vi "Main_State.vi"() -> ()   [LabVIEW 2017]
doc: "This sample project is built upon the standard state machine template and shows how you could create an application that acquires, analyzes, and presents data. It includes functionality for presenting configuration dialogs, preserving settings between executions, loading and saving data, as well as exporting graph images and text files.\n\nIt is most appropriate for data that is acquired instantly as it does not allow for screen updates mid acquisition nor does it allow for continuous streaming to disk."
uses:
  controls/State.ctl
  controls/Data.ctl
  controls/UI References.ctl
  controls/User Specified Data.ctl
  controls/HW Configuration.ctl
  controls/Analysis Configuration.ctl
  controls/New Data Behavior.ctl
  controls/Signal Configuration.ctl
  controls/TCP Multiple Connections State.ctl
  controls/TCP Multiple Connections Data.ctl
  <extravilib>/ChannelInstances/Event Messenger-str/Instantiate.vi
  <extravilib>/ChannelInstances/Event Messenger-str/))Channel.vi
  <extravilib>/ChannelInstances/Event Messenger-c(a[.](str),t'Data.ctl')/Instantiate.vi
  <extravilib>/ChannelInstances/Event Messenger-c(a[.](str),t'Data.ctl')/))Channel.vi
  subVIs/Settings Dialog.vi
  <extravilib>/ChannelInstances/Event Messenger-str.lvlib
  <extravilib>/ChannelInstances/Event Messenger-c(a[.](str),t'Data.ctl').lvlib
panel:
  out "# of Connections":i32
  in  "Settings":bool
  in  "Snapshot":bool
  in  "Analyze":bool
  in  "Clear":bool
  in  "Exit":bool
  in  "Acquire":bool
  in  "Export":bool
  in  "Save Data":bool
  in  "Load Data":bool
  out "Status Bar":string
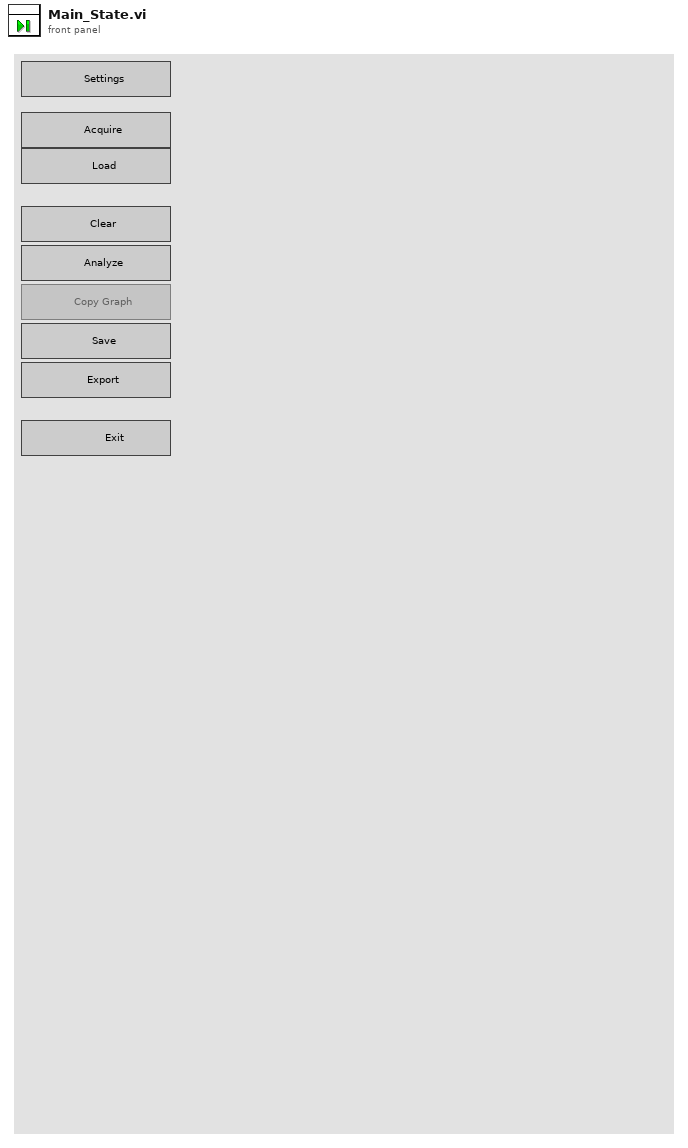
[diagram p1: front panel]
types:
  T1 = typedef "TCP Multiple Connections Data.ctl" = cluster{"Clients":refnum<k5>[], "Listener":refnum<k5>}
  T2 = typedef "TCP Multiple Connections State.ctl" = enum16{"Initialize", "Status Check", "Send Data", "Stop"}
  T3 = typedef "Data.ctl" = cluster{"UI References":T4, "User Specified":T5}
  T4 = typedef "UI References.ctl" = cluster{"Exit Ref":refnum<vi>, "Save Ref":refnum<vi>, "Open Ref":refnum<vi>, "Export Ref":refnum<vi>, "Acquire Ref":refnum<vi>, "Configure Ref":refnum<vi>, "Graph Ref":refnum<vi>, "Clear Ref":refnum<vi>, "Analyze Ref":refnum<vi>, "Status Ref":refnum<vi>, "Snapshot Ref":refnum<vi>}
  T5 = typedef "User Specified Data.ctl" = cluster{"Hardware Configuration":T6, "Analysis Configuration":T7, "Signal Type":enum16{"Single Chirp", "From Excel"}, "New Data Behavior":T8, "Signal Configuration":T9, "Waveform File":string, "Save Location":string}
  T6 = typedef "HW Configuration.ctl" = cluster{"Signal Channel":tag, "Response Channel":tag, "Trigger Channel":tag, "Number of Acquisitions":dbl}
  T7 = typedef "Analysis Configuration.ctl" = cluster{"Statistics":bool}
  T8 = typedef "New Data Behavior.ctl" = enum16{"Replace", "Overlay", "Append"}
  T9 = typedef "Signal Configuration.ctl" = cluster{"Chirp Amplitude":dbl, "I/O Limit":dbl, "Sample Rate":dbl, "Chirp Duration (s)":dbl, "Upper Frequency":dbl, "Lower Frequency":dbl, "Windowing":enum16{"None", "Exponential", "Flat top", "Hamming", "Hanning", "Kaiser-Bessel", "Rectangular"}}
  T10 = typedef "State.ctl" = enum16{"Initialize", "Wait for Event", "Update UI", "Configure", "Acquire", "Load Data", "Save Data", "Clear Data", "Export Data", "Analyze", "Copy Graph", "Exit"}
  T11 = enum16{"Standard", "Buffered", "CRLF", "Immediate"}
  T12 = typedef "Event Messenger-str.lvlib/))Channel.ctl" = refnum<queue>
  T13 = cluster{"Event message":string[], "User Specified Data":T3}
  T14 = typedef "Event Messenger-c(a[.](str),t'Data.ctl').lvlib/))Channel.ctl" = refnum<queue>
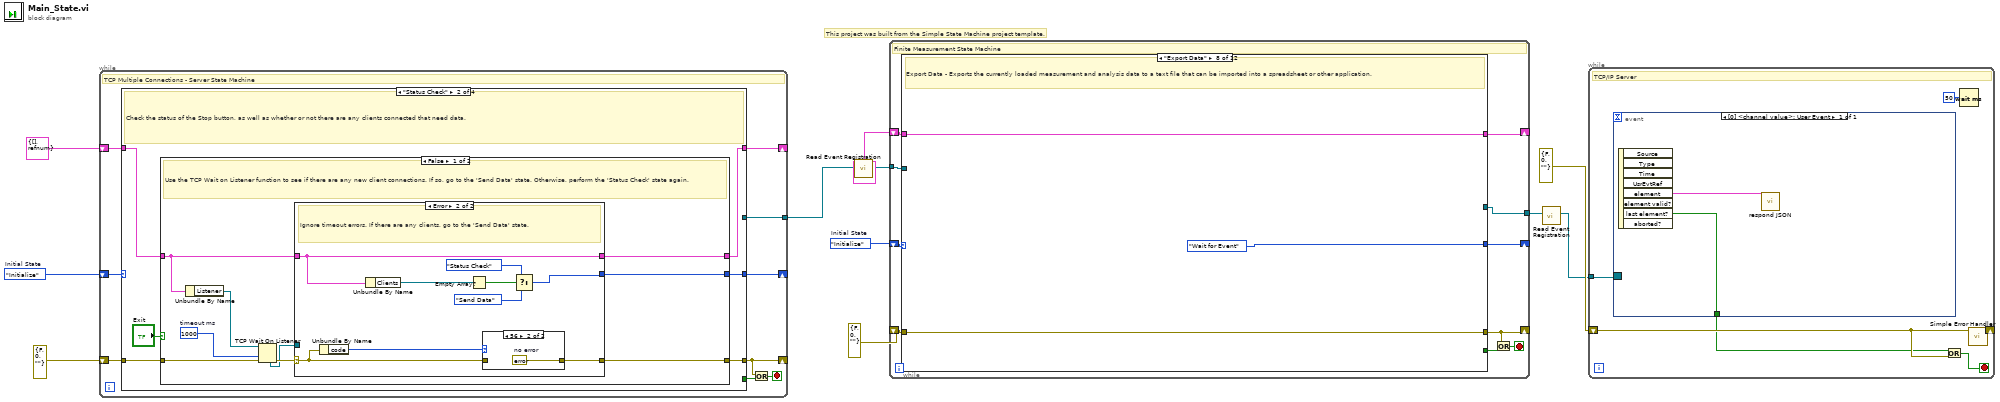
[diagram p0: block diagram]
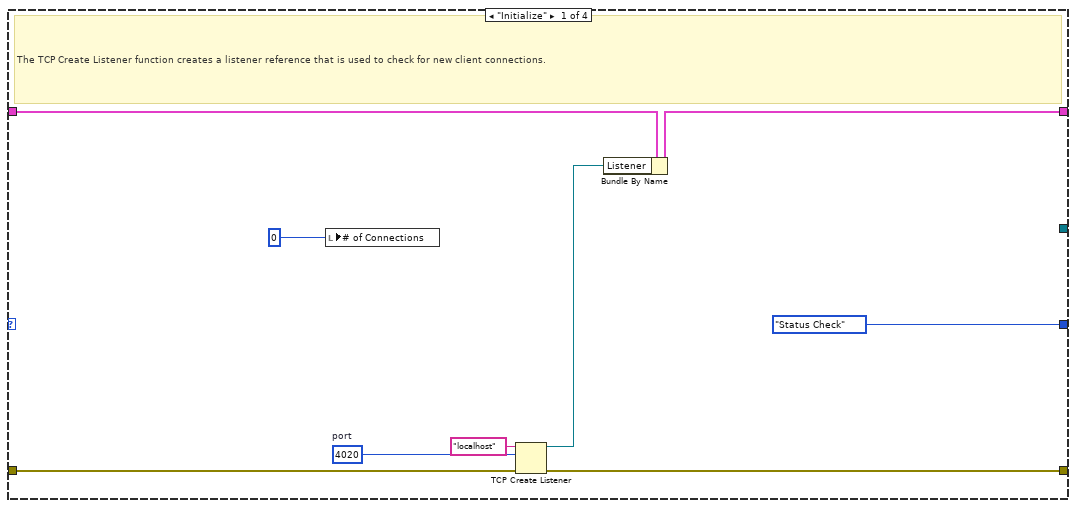
[diagram p2: hidden frame]
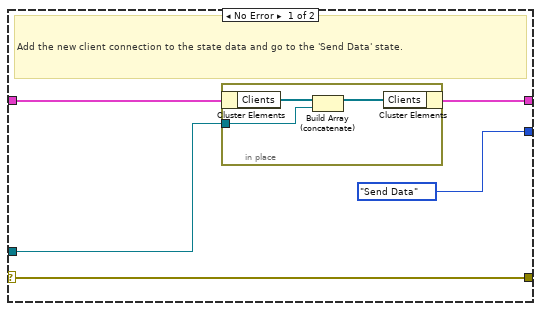
[diagram p3: hidden frame]
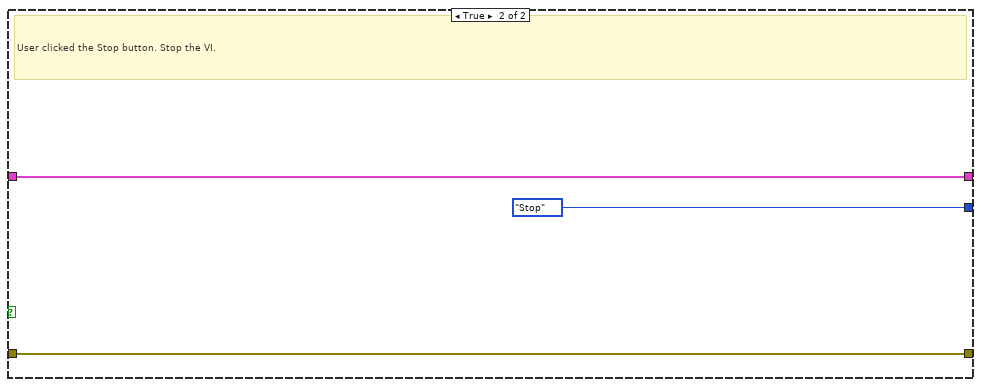
[diagram p5: hidden frame]
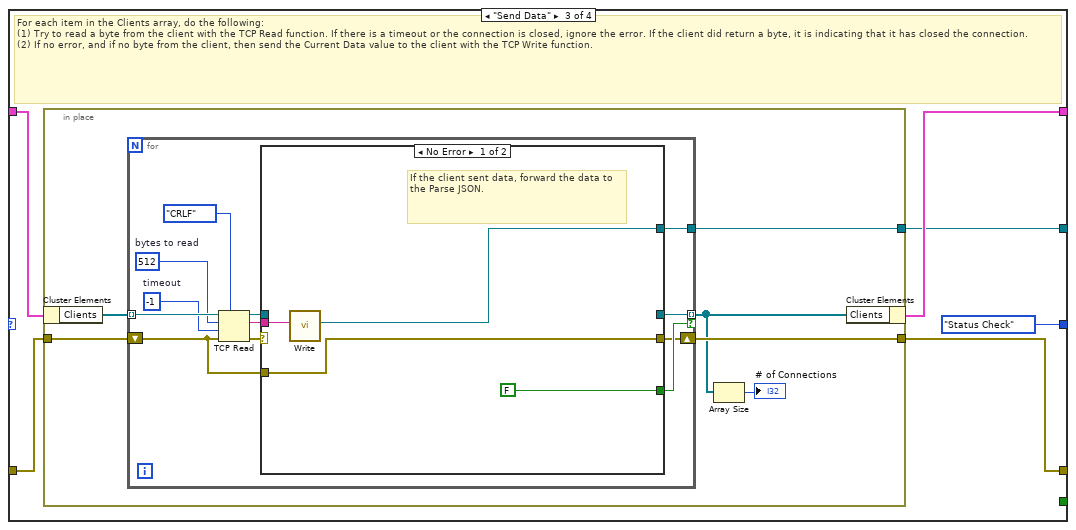
[diagram p6: hidden frame]
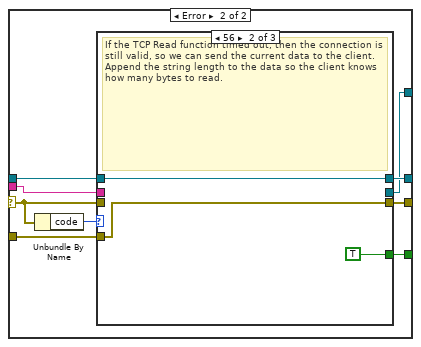
[diagram p7: hidden frame]
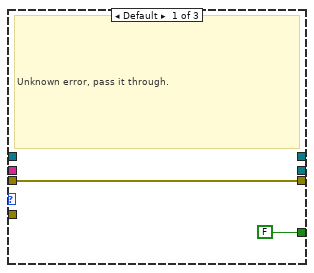
[diagram p8: hidden frame]
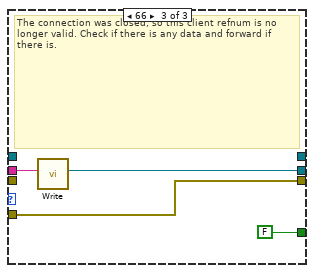
[diagram p9: hidden frame]
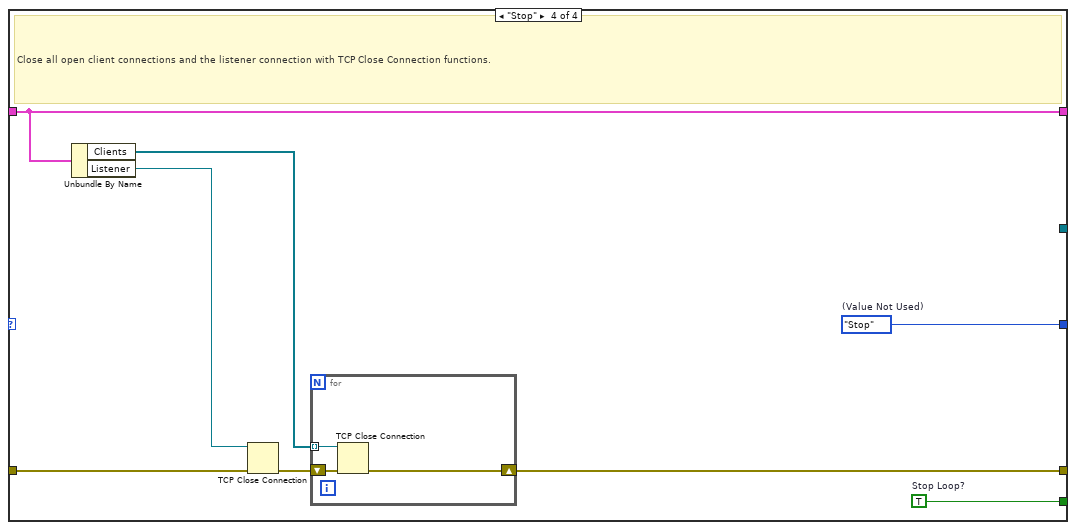
[diagram p10: hidden frame]
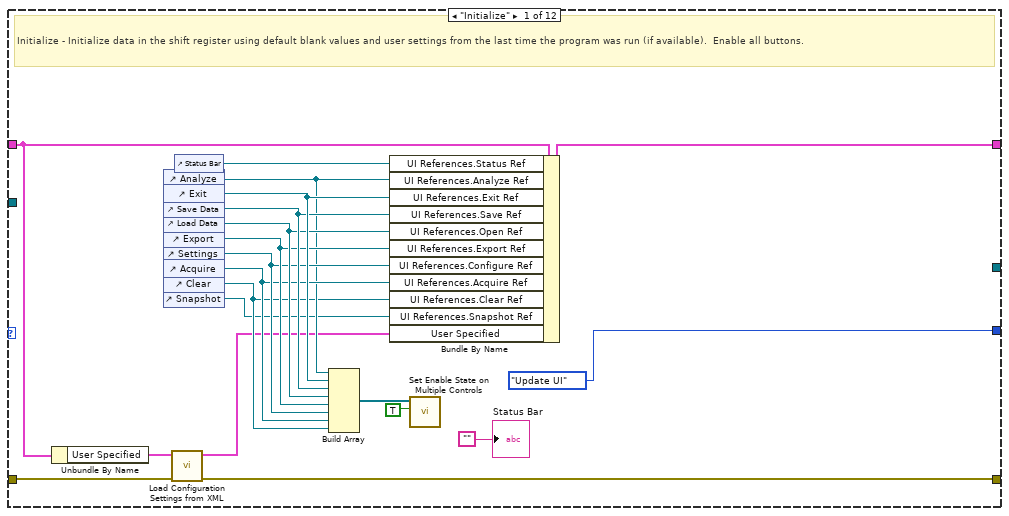
[diagram p11: hidden frame]
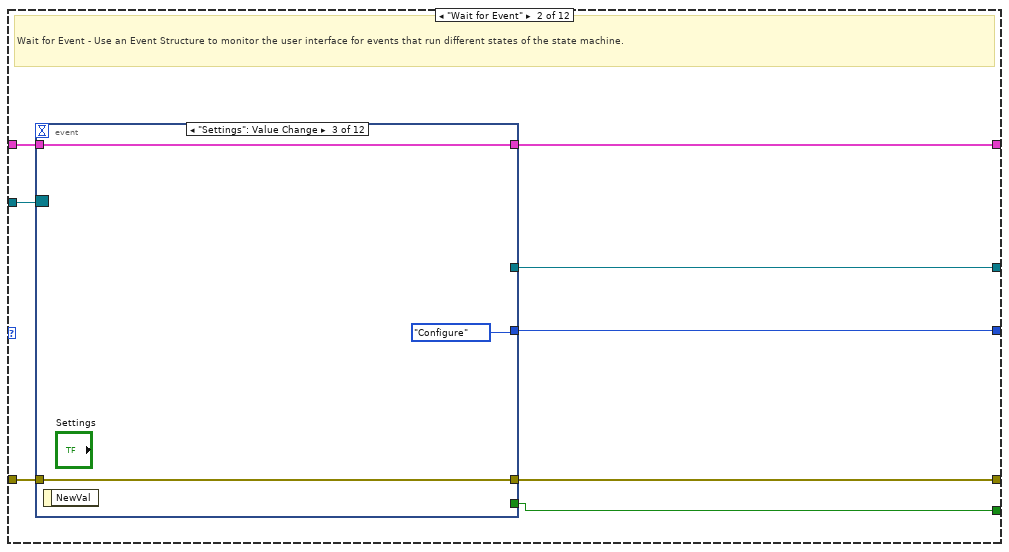
[diagram p12: hidden frame]
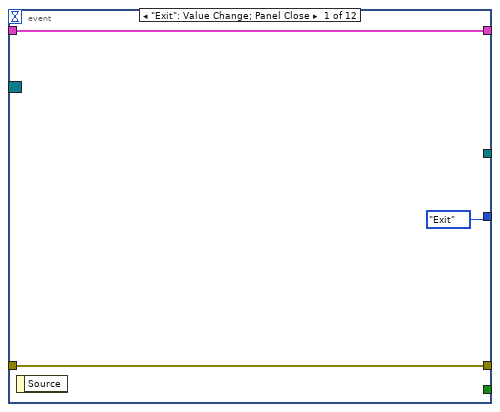
[diagram p13: hidden frame]
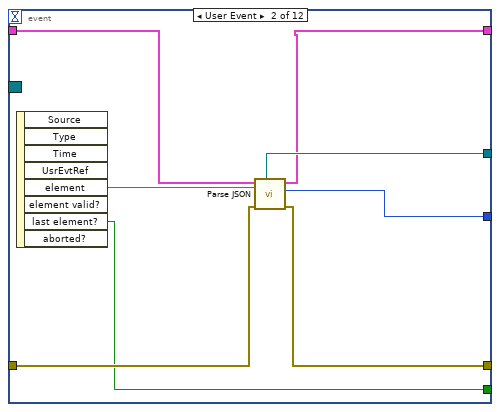
[diagram p14: hidden frame]
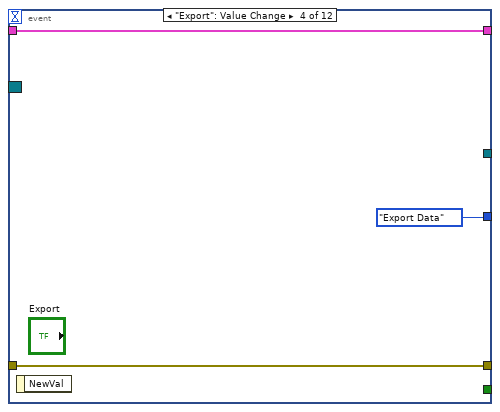
[diagram p15: hidden frame]
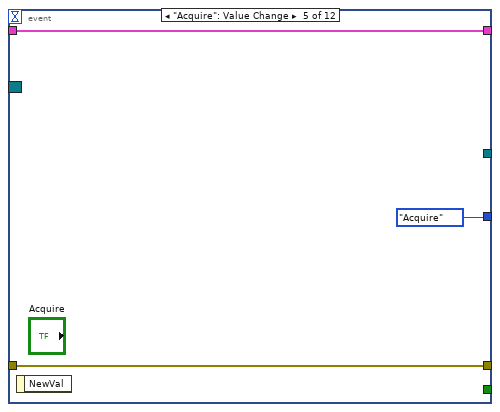
[diagram p16: hidden frame]
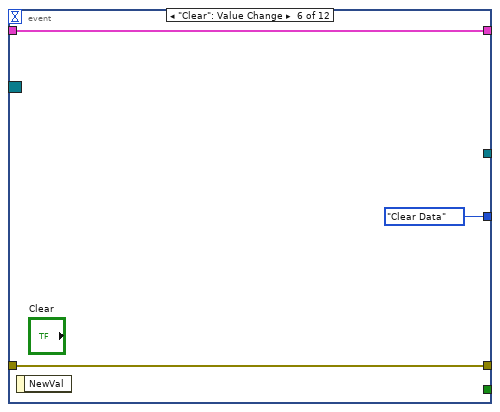
[diagram p17: hidden frame]
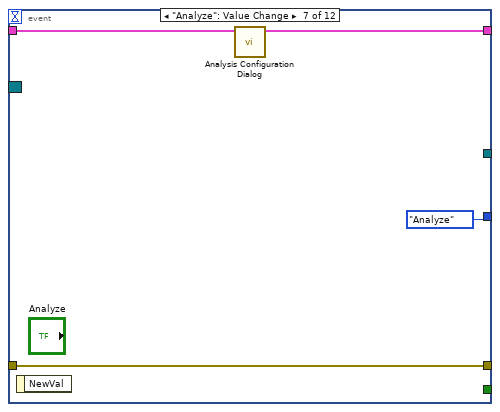
[diagram p18: hidden frame]
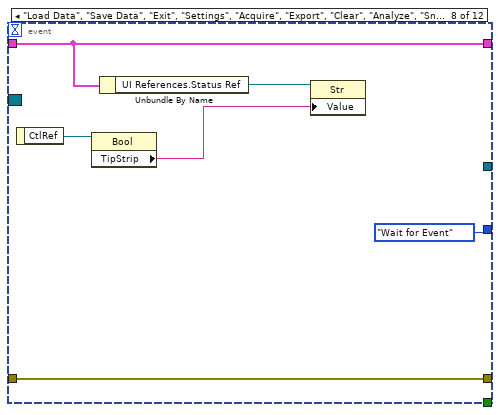
[diagram p19: hidden frame]
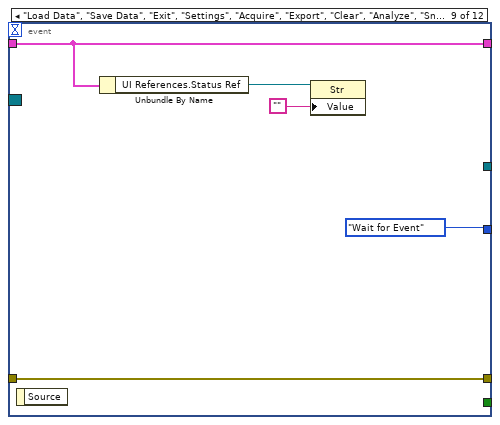
[diagram p20: hidden frame]
diagram:
  w4 = TCP_Multiple_Connections_State."Initialize"  # Initial State
  w11 = State."Initialize"  # Initial State
  # "This project was built from the Simple State Machine project template."
  n1 = while {
    shift-right: [w19] -> _
    shift-left: w4 -> [w20]
    shift-right: [w17] -> _
    shift-left: T1 {"Clients"=[], "Listener"=refnum} ("Data") -> [w18]
    shift-right: [w13] -> _
    shift-left: errorcluster {"status"=FALSE, "code"=0, "source"=""} ("error constant") -> [w16]
    tunnel: [w12] -> w1
    stop <- w14 stop-if-true
    # "TCP Multiple Connections - Server State Machine"
    n2 = case shown="\"Status Check\"" w20 {
      tunnel: [TCP_Multiple_Connections_State."Status Check" ("States") w35 TCP_Multiple_Connections_State."Status Check" ("States") w113] -> w19
      tunnel: [_ _ _ w120] -> w15
      tunnel: w18 -> [w27 w32 w70 w119]
      tunnel: [w26 w31 w69 w119] -> w17
      tunnel: w16 -> [w29 w34 w72 w118]
      tunnel: [w28 w33 w71 w116] -> w13
      tunnel: [_ _ w67 _] -> w12
      frame "Initialize" {
        w24 = u16 4020  # port
        # "The TCP Create Listener function creates a listener reference that is used to check for new client connections."
        n3 = local write "# of Connections"(0 ("Number of Client Connections")) -> ()
        n4 = TCP Create Listener(8:w29, 10:w24, 11:"localhost" ("service name")) -> (0:w28:errorcluster, 3:w25:refnum<k5>)  [unwired: 3 out]
        n5 = Bundle By Name(cluster=w27, "Listener"=w25) -> (w26:T1)
      }
      frame "Status Check" {
        # "Check the status of the Stop button, as well as whether or not there are any clients connected that need data."
        n6 = case shown="False" "Exit" {
          tunnel: [w44 TCP_Multiple_Connections_State."Stop" ("States")] -> w35
          tunnel: w34 -> [w43 w66]
          tunnel: [w36 w66] -> w33
          tunnel: w32 -> [w39 w65]
          tunnel: [w38 w65] -> w31
          frame False {
            w42 = 1000  # timeout ms
            # "Use the TCP Wait on Listener function to see if there are any new client connections. If so, go to the 'Send Data' state. Otherwise, perform the 'Status Check' state again."
            n7 = Unbundle By Name(w39) -> ("Listener"=w37:refnum<k5>)
            n8 = TCP Wait On Listener(8:w43, 9:w42, 11:w37) -> (0:w41:errorcluster, 4:w40:refnum<k5>)  [unwired: 4 out]
            n9 = case shown="Error" w41 {
              selector: w41 -> [w47 w61]
              tunnel: [TCP_Multiple_Connections_State."Send Data" ("States") w55] -> w44
              tunnel: w40 -> [w48 _]
              tunnel: w39 -> [w49 w58]
              tunnel: [w46 w58] -> w38
              tunnel: [w47 w59] -> w36
              frame No Error {
                # "Add the new client connection to the state data and go to the 'Send Data' state."
                n10 = in-place {
                  in-place-border: w48 -> [w50]
                  n11 = in-place-cluster #1(w49) -> ("Clients"=w52:refnum<k5>[])
                  n12 = Build Array (concatenate)(w52, w50) -> (w51:refnum<k5>[])
                  n13 = in-place-cluster #1("Clients"=w51) -> (w46:T1)
                }
              }
              frame Error {
                # "Ignore timeout errors. If there are any clients, go to the 'Send Data' state."
                n14 = Unbundle By Name(w61) -> ("code"=w60:i32)
                n15 = Unbundle By Name(w58) -> ("Clients"=w57:refnum<k5>[])
                n16 = Empty Array?(array=w57) -> (empty?=w56:bool)
                n17 = case shown="56" w60 {
                  tunnel: w61 -> [w62 _]
                  tunnel: [w62 w63] -> w59
                  frame Default {
                  }
                  frame 56 {
                    w63 = errorcluster {"status"=FALSE, "code"=0, "source"=""}  # no error
                  }
                }
                n18 = Select(t=TCP_Multiple_Connections_State."Status Check" ("States"), s=w56, f=TCP_Multiple_Connections_State."Send Data" ("States")) -> (s? t:f=w55:T2)
              }
            }
          }
          frame True {
            # "User clicked the Stop button. Stop the VI."
          }
        }
      }
      frame "Send Data" {
        # "For each item in the Clients array, do the following:\n(1) Try to read a byte from the client with the TCP Read function. If there is a timeout or the connection is closed, ignore the error. If the client did return a byte, it is indicating that it has closed the connection.\n(2) If no error, and if no byte from the client, then send the Current Data value to the client with the TCP Write function."
        n19 = in-place {
          in-place-border: w72 -> [w78]
          in-place-border: [w77] -> w71
          in-place-border: [w73] -> w67
          n20 = in-place-cluster #2(w70) -> ("Clients"=w75:refnum<k5>[])
          n21 = for {
            tunnel: w75 -> [w90] mode=indexing
            shift-right: [w82] -> w77
            shift-left: w78 -> [w81]
            tunnel: [w84] -> w74 mode=indexing if=w83
            tunnel: [w79] -> w73
            w87 = -1  # timeout
            w88 = 512  # bytes to read
            n22 = TCP Read(connection ID=w90, bytes to read=w88, error in (no error)=w81, 7:T11."CRLF" ("mode (standard)"), 9:w87) -> (connection ID out=w89:refnum<k5>, data out=w85:string, error out=w86:errorcluster)
            n23 = case shown="No Error" w86 {
              selector: w86 -> [_ w102]
              tunnel: w89 -> [_ w99]
              tunnel: w85 -> [w91 w96]
              tunnel: [_ w97] -> w84
              tunnel: [FALSE w98] -> w83
              tunnel: [w92 w101] -> w82
              tunnel: w81 -> [w92 w100]
              tunnel: [w93 w95] -> w79
              frame No Error {
                # "If the client sent data, forward the data to the Parse JSON."
                # "If the client sent data, it is saying that the connection should be closed."
                n24 = call <extravilib>:"Write.vi"("element"=w91) -> ("channel"=w93:T12)  [unwired: 9 in, 1 out]
              }
              frame Error {
                # "Ignore connection closed and timeout errors"
                n25 = Unbundle By Name(w102) -> ("code"=w103:i32)
                n26 = case shown="56" w103 {
                  tunnel: w102 -> [w105 _ _]
                  tunnel: [w105 w106 w112] -> w101
                  tunnel: w100 -> [_ w106 w112]
                  tunnel: w99 -> [_ w108 _]
                  tunnel: [FALSE TRUE FALSE] -> w98
                  tunnel: [_ w108 _] -> w97
                  tunnel: w96 -> [_ _ w110]
                  tunnel: [_ _ w109] -> w95
                  frame Default {
                    # "Unknown error, pass it through."
                  }
                  frame 56 {
                    # "If the TCP Read function timed out, then the connection is still valid, so we can send the current data to the client. Append the string length to the data so the client knows how many bytes to read."
                  }
                  frame 66 {
                    # "The connection was closed, so this client refnum is no longer valid. Check if there is any data and forward if there is."
                    n27 = call <extravilib>:"Write.vi"("element"=w110) -> ("channel"=w109:T12)  [unwired: 9 in, 1 out]
                  }
                }
              }
            }
          }
          n28 = Array Size(array=w74) -> (size(s)=→"# of Connections":i32)
          n29 = in-place-cluster #2("Clients"=w74) -> (w69:T1)
        }
      }
      frame "Stop" {
        w113 = TCP_Multiple_Connections_State."Stop"  # (Value Not Used)
        w120 = TRUE  # Stop Loop?
        # "Close all open client connections and the listener connection with TCP Close Connection functions."
        n30 = Unbundle By Name(w119) -> ("Clients"=w117:refnum<k5>[], "Listener"=w114:refnum<k5>)
        n31 = TCP Close Connection(connection ID=w114, error in (no error)=w118) -> (error out=w115:errorcluster)  [unwired: 1 in, 1 out]
        n32 = for {
          shift-right: [w122] -> w116
          shift-left: w115 -> [w123]
          tunnel: w117 -> [w121] mode=indexing
          n33 = TCP Close Connection(connection ID=w121, error in (no error)=w123) -> (error out=w122:errorcluster)  [unwired: 1 in, 1 out]
        }
      }
    }
    n34 = Or(x=w13, y=w15) -> (x .or. y?=w14:bool)
  }
  n35 = call <extravilib>:"Read Event Registration.vi"("channel"=w1) -> ("event registration refnum"=w9:refnum<event-registration>)  [unwired: 10 in]
  n36 = while {
    shift-right: [w125] -> _
    shift-left: w11 -> [w133]
    shift-right: [w131] -> _
    shift-left: T3 {"UI References"={"Exit Ref"=refnum, "Save Ref"=refnum, "Open Ref"=refnum, "Export Ref"=refnum, "Acquire Ref"=refnum, "Configure Ref"=refnum, "Graph Ref"=refnum, "Clear Ref"=refnum, "Analyze Ref"=refnum, "Status Ref"=refnum, "Snapshot Ref"=refnum}, "User Specified"={"Hardware Configuration"={"Signal Channel"="", "Response Channel"="", "Trigger Channel"="", "Number of Acquisitions"=0.0}, "Analysis Configuration"={"Statistics"=TRUE}, "Signal Type"=enum."Single Chirp", "New Data Behavior"=enum."Replace", "Signal Configuration"={"Chirp Amplitude"=0.1, "I/O Limit"=10.0, "Sample Rate"=1000000.0, "Chirp Duration (s)"=0.01, "Upper Frequency"=0.0, "Lower Frequency"=0.0, "Windowing"=enum."None"}, "Waveform File"="", "Save Location"=""}} ("Data") -> [w132]
    shift-right: [w128] -> _
    shift-left: errorcluster {"status"=FALSE, "code"=0, "source"=""} ("error constant") -> [w130]
    tunnel: w9 -> [w127]
    tunnel: [w126] -> w6
    stop <- w124 stop-if-true
    # "Finite Measurement State Machine"
    n37 = case shown="\"Export Data\"" w133 {
      tunnel: [_ w161 _ _ _ _ _ _ _ _ _ w265] -> w126
      tunnel: [_ w154 _ _ _ _ _ _ _ _ _ w276] -> w129
      tunnel: w132 -> [w145 w160 w210 w221 w224 w241 w249 w253 w254 w258 w263 w274]
      tunnel: [w153 w159 w210 w220 w225 w238 w249 w253 w254 w258 w263 w274] -> w131
      tunnel: w130 -> [w143 w158 w211 w219 w228 w235 w248 w251 w256 w259 w262 w271]
      tunnel: [w142 w157 w211 w218 w228 w240 w248 w251 w256 w259 w261 w270] -> w128
      tunnel: w127 -> [_ w156 _ _ _ _ _ _ _ _ _ _]
      tunnel: [State."Update UI" ("Next State") w155 State."Wait for Event" ("(Value Not Used)") w212 State."Update UI" ("Next State") State."Update UI" ("(Value Not Used)") State."Wait for Event" ("(Value Not Used)") State."Wait for Event" ("(Value Not Used)") State."Update UI" ("(Value Not Used)") State."Update UI" ("(Value Not Used)") State."Wait for Event" ("(Value Not Used)") w269] -> w125
      frame "Initialize" {
        # "Initialize - Initialize data in the shift register using default blank values and user settings from the last time the program was run (if available).  Enable all buttons."
        n38 = Unbundle By Name(w145) -> ("User Specified"=w144:T5)
        n39 = control-ref of="Analyze"() -> (w141:refnum<vi>)
        n40 = control-ref of="Exit"() -> (w152:refnum<vi>)
        n41 = control-ref of="Save Data"() -> (w151:refnum<vi>)
        n42 = control-ref of="Load Data"() -> (w150:refnum<vi>)
        n43 = control-ref of="Export"() -> (w149:refnum<vi>)
        n44 = control-ref of="Settings"() -> (w148:refnum<vi>)
        n45 = control-ref of="Acquire"() -> (w147:refnum<vi>)
        n46 = control-ref of="Clear"() -> (w139:refnum<vi>)
        n47 = control-ref of="Snapshot"() -> (w135:refnum<vi>)
        n48 = call "Load Configuration Settings from XML.vi"("error in (no error)"=w143, "User Configuration in"=w144) -> ("error out"=w142:errorcluster, "User Configuration out"=w137:T5)  [unwired: 8 in]
        n49 = control-ref of="Status Bar"() -> (w140:refnum<vi>)
        n50 = Build Array(w141, w152, w151, w150, w149, w148, w147, w139) -> (w146:refnum<vi>[])
        n51 = Bundle By Name(cluster=w145, "UI References.Status Ref"=w140, "UI References.Analyze Ref"=w141, "UI References.Exit Ref"=w152, "UI References.Save Ref"=w151, "UI References.Open Ref"=w150, "UI References.Export Ref"=w149, "UI References.Configure Ref"=w148, "UI References.Acquire Ref"=w147, "UI References.Clear Ref"=w139, "UI References.Snapshot Ref"=w135, "User Specified"=w137) -> (w153:T3)
        n52 = call "Set Enable State on Multiple Controls.vi"("Enable?"=TRUE, "Controls"=w146) -> ()  [unwired: 10 in]
        "Status Bar" <- "" ("Status Bar")
      }
      frame "Wait for Event" {
        # "Wait for Event - Use an Event Structure to monitor the user interface for events that run different states of the state machine."
        n53 = event shown="[2] \"Settings\": Value Change" {
          selector: w156 -> [_ _ _ _ _ _ _ _ _ _ _ _]
          dyn-events: _ -> [_ _ _ _ _ _ _ _ _ _ _ _]
          timeout: _ -> [_ _ _ _ _ _ _ _ _ _ _ _]
          tunnel: [_ w168 _ _ _ _ _ _ _ _ _ _] -> w161
          tunnel: w160 -> [w164 w171 w175 w178 w181 w184 w187 w192 w198 w202 w205 w208]
          tunnel: [w164 w166 w175 w178 w181 w184 w186 w192 w198 w202 w205 w208] -> w159
          tunnel: w158 -> [w163 w170 w174 w177 w180 w183 w188 w194 w199 w201 w204 w207]
          tunnel: [w163 w169 w174 w177 w180 w183 w188 w194 w199 w201 w204 w207] -> w157
          tunnel: [State."Exit" ("Next State") w167 State."Configure" ("Next State") State."Export Data" ("Next State") State."Acquire" ("Next State") State."Clear Data" ("Next State") State."Analyze" ("Next State") State."Wait for Event" ("Next State") State."Wait for Event" ("Next State") State."Copy Graph" ("Next State") State."Load Data" ("Next State") State."Save Data" ("Next State")] -> w155
          tunnel: [_ w165 _ _ _ _ _ _ _ _ _ _] -> w154
          event "Exit": Value Change; Panel Close {
            n54 = event-data() -> ()  [unwired: 1 in, 1 out]
          }
          event User Event {
            n55 = event-data() -> ("element"=w172:string, "last element?"=w165:bool)  [unwired: 1 in, 6 out]
            n56 = call "Parse JSON.vi"("error in (no error)"=w170, "element"=w172, "Data In"=w171) -> ("error out"=w169:errorcluster, "States"=w167:T10, "Data Out"=w166:T3, "channel"=w168:T14)  [unwired: 3 in]
          }
          event "Settings": Value Change {
            n57 = event-data() -> ()  [unwired: 1 in, 1 out]
          }
          event "Export": Value Change {
            n58 = event-data() -> ()  [unwired: 1 in, 1 out]
          }
          event "Acquire": Value Change {
            n59 = event-data() -> ()  [unwired: 1 in, 1 out]
          }
          event "Clear": Value Change {
            n60 = event-data() -> ()  [unwired: 1 in, 1 out]
          }
          event "Analyze": Value Change {
            n61 = event-data() -> ()  [unwired: 1 in, 1 out]
            n62 = call "Analysis Configuration Dialog.vi"("Data in"=w187) -> ("Data out"=w186:T3)  [unwired: 10 in]
          }
          event "Load Data", "Save Data", "Exit", "Settings", "Acquire", "Export", "Clear", "Analyze", "Snapshot": Mouse Enter {
            n63 = event-data() -> ("CtlRef"=w193:refnum<vi>)  [unwired: 1 in]
            n64 = property class="Bool"(reference=w193) -> ("TipStrip"=w190:string)  [unwired: 1 in, 2 out]
            n65 = Unbundle By Name(w192) -> ("UI References.Status Ref"=w191:refnum<vi>)
            n66 = property class="Str"(reference=w191, "Value"=w190) -> ()  [unwired: 1 in, 2 out]
          }
          event "Load Data", "Save Data", "Exit", "Settings", "Acquire", "Export", "Clear", "Analyze", "Snapshot": Mouse Leave {
            n67 = event-data() -> ()  [unwired: 1 in, 1 out]
            n68 = Unbundle By Name(w198) -> ("UI References.Status Ref"=w197:refnum<vi>)
            n69 = property class="Str"(reference=w197, "Value"="") -> ()  [unwired: 1 in, 2 out]
          }
          event "Snapshot": Value Change {
            n70 = event-data() -> ()  [unwired: 1 in, 1 out]
          }
          event "Load Data": Value Change {
            n71 = event-data() -> ()  [unwired: 1 in, 1 out]
          }
          event "Save Data": Value Change {
            n72 = event-data() -> ()  [unwired: 1 in, 1 out]
          }
        }
      }
      frame "Update UI" {
        # "Update UI - Update the graph using the waveform data stored in the shift register.  If there is no data to display disable buttons that act on the current data."
      }
      frame "Configure" {
        # "Configure - Spawns a dialog that allows the user to set any user configurable settings."
        n73 = Unbundle By Name(w221) -> ("User Specified"=w214:T5)
        n74 = call-by-ref "?"("error in (no error)"=w219, "Configuration in"=w214) -> ("error out"=w218:errorcluster, "UI Refresh Needed?"=w217:bool, "Configuration out"=w213:T5)  [unwired: 9 in, 2 out]
        n75 = Bundle By Name(cluster=w221, "User Specified"=w213) -> (w220:T3)
        n76 = Select(t=State."Update UI" ("Next State if true"), s=w217, f=State."Wait for Event" ("Next State if false")) -> (s? t:f=w212:T10)
      }
      frame "Acquire" {
        # "Acquire - Uses the current hardware configuration to acquire a new data set and stores it in the state data."
        n77 = Unbundle By Name(w224) -> ("UI References.Status Ref"=w226:refnum<vi>, "User Specified"=w223:T5)  [unwired: 1 out]
        n78 = call "Acquire Data from Hardware N times.vi"("User Specified"=w223) -> ("error out"=w222:errorcluster)  [unwired: 9 in]
        n79 = case shown="No Error" w222 {
          selector: w222 -> [_ w234]
          tunnel: [w230 w232] -> w225
          tunnel: ["Data acquired." ("Data acquired") "Data not acquired." ("Data not acquired")] -> w227
          tunnel: w224 -> [w230 w232]
          frame No Error {
          }
          frame Error {
            n80 = call <vilib>:"Simple Error Handler.vi"("error in (no error)"=w234) -> ()  [unwired: 4 in, 5 out]
          }
        }
        n81 = property class="Str"(reference=w226, "Value"=w227) -> ()  [unwired: 1 in, 2 out]
      }
      frame "Load Data" {
        # "Load Data - Loads data from a TDMS file and incorporates it with the existing data according to the user's preference."
        n82 = case shown="No Error" w235 {
          selector: w235 -> [w242 w246]
          tunnel: w241 -> [w243 w247]
          tunnel: [w243 w247] -> w238
          tunnel: [w242 _] -> w240
          tunnel: ["Data loaded." ("Data loaded") "Data not loaded." ("Data not loaded")] -> w239
          frame No Error {
          }
          frame Error {
            n83 = call <vilib>:"Simple Error Handler.vi"("error in (no error)"=w246) -> ()  [unwired: 4 in, 5 out]
          }
        }
        n84 = Unbundle By Name(w238) -> ("UI References.Status Ref"=w237:refnum<vi>)
        n85 = property class="Str"(reference=w237, "Value"=w239) -> ()  [unwired: 1 in, 2 out]
      }
      frame "Save Data" {
        # "Save Data - Saves the existing measurement data to a TDMS file."
      }
      frame "Export Data" {
        # "Export Data - Exports the currently loaded measurement and analysis data to a text file that can be imported into a spreadsheet or other application."
      }
      frame "Clear Data" {
        # "Clear Data - Clears the data currently in the graph."
      }
      frame "Analyze" {
        # "#CodeRecommended - Add your own signal analysis here."
        # "Analyze - Analyzes the measurement data."
      }
      frame "Copy Graph" {
        # "Copy Graph - Places an image of the graph on the clipboard for pasting into reports or emails."
        n86 = call "Copy Graph to Clipboard.vi"("error in (no error)"=w262, "Graph Data"=w263) -> ("error out"=w261:errorcluster)  [unwired: 9 in]
      }
      frame "Exit" {
        w276 = TRUE  # Stop Loop?
        w269 = State."Exit"  # (Value Not Used)
        # "Exit - Saves the user's settings to an XML file and stops execution."
        n87 = Unbundle By Name(w274) -> ("UI References.Status Ref"=w272:refnum<vi>, "User Specified"=w275:T5)
        n88 = call "Save Configuration Settings to XML.vi"("error in (no error)"=w271, "User Configuration"=w275) -> ("error out"=w270:errorcluster)  [unwired: 9 in]
        n89 = property class="Str"(reference=w272, "Value"="Application exit." ("Stopped")) -> ()  [unwired: 1 in, 2 out]
        n90 = Bundle By Name(cluster=T13 {"Event message"=[], "User Specified Data"={"UI References"={"Exit Ref"=refnum, "Save Ref"=refnum, "Open Ref"=refnum, "Export Ref"=refnum, "Acquire Ref"=refnum, "Configure Ref"=refnum, "Graph Ref"=refnum, "Clear Ref"=refnum, "Analyze Ref"=refnum, "Status Ref"=refnum, "Snapshot Ref"=refnum}, "User Specified"={"Hardware Configuration"={"Signal Channel"="", "Response Channel"="", "Trigger Channel"="", "Number of Acquisitions"=0.0}, "Analysis Configuration"={"Statistics"=TRUE}, "Signal Type"=enum."Single Chirp", "New Data Behavior"=enum."Replace", "Signal Configuration"={"Chirp Amplitude"=10.0, "I/O Limit"=10.0, "Sample Rate"=1000000.0, "Chirp Duration (s)"=0.01, "Upper Frequency"=0.0, "Lower Frequency"=0.0, "Windowing"=enum."None"}, "Waveform File"="", "Save Location"=""}}}, "Event message"=string[] ["experimentStopped"]) -> (w266:T13)
        n91 = call <extravilib>:"Write.vi"("last element? (F)"=TRUE, "element"=w266) -> ("channel"=w265:T14)  [unwired: 8 in, 1 out]
      }
    }
    n92 = Or(x=w128, y=w129) -> (x .or. y?=w124:bool)
  }
  n93 = call <extravilib>:"Read Event Registration.vi"("channel"=w6) -> ("event registration refnum"=w5:refnum<event-registration>)  [unwired: 10 in]
  n94 = while {
    shift-right: [w278] -> _
    shift-left: errorcluster {"status"=FALSE, "code"=0, "source"=""} ("error constant") -> [w278]
    tunnel: w5 -> [w281]
    stop <- w279 stop-if-true
    # "TCP/IP Server"
    n95 = event shown="[0] <channel value>: User Event" {
      selector: w281 -> [_]
      dyn-events: _ -> [_]
      timeout: _ -> [_]
      tunnel: [w282] -> w277
      event User Event {
        n96 = event-data() -> ("element"=w283:cluster{string[], "Data In 2":T3}, "last element?"=w282:bool)  [unwired: 1 in, 6 out]
        n97 = call "respond JSON.vi"("Message In"=w283) -> ()  [unwired: 11 in]
      }
    }
    n98 = Or(x=w277, y=w278) -> (x .or. y?=w279:bool)
    n99 = Wait (ms)(milliseconds to wait=u32 50) -> ()  [unwired: 1 out]
  }
  n100 = call <vilib>:"Simple Error Handler.vi"() -> ()  [unwired: 5 in, 5 out]
